vi "GetFilterList.vi"(11 "Templates":refnum<class "MetaDataObj.lvclass">[](array[class])) -> (3 "Filters":string[](array[string]))   [LabVIEW 2016, in "NI_NPW_Filters.lvlib"]
uses:
  <resource>/dialog/NewProjectWizard/Filters/NI_NPW_Filters.lvlib
  <resource>/dialog/NewProjectWizard/MetaDataObj/MetaDataObj.lvclass
  <resource>/dialog/NewProjectWizard/MetaDataObj/Accessors/Read Filters.vi
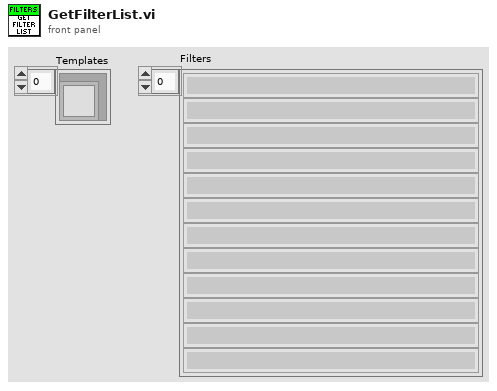
[diagram p1: front panel]
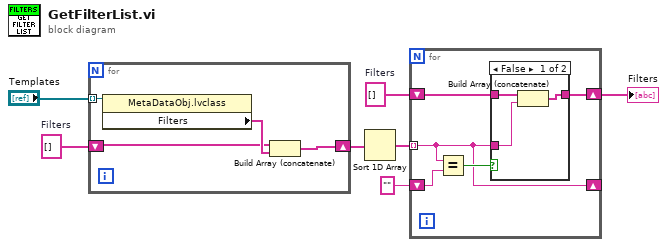
[diagram p0: block diagram]
diagram:
  w4 = string[] []  # Filters
  w6 = string[] []  # Filters
  n1 = for {
    tunnel: "Templates" -> [w11] mode=indexing
    shift-right: [w8] -> w5
    shift-left: w6 -> [w9]
    n2 = property class="MetaDataObj.lvclass"(reference=w11) -> ("Filters"=w10:string[])  [unwired: 1 in, 2 out]
    n3 = Build Array (concatenate)(w9, w10) -> (w8:string[])
  }
  n4 = Sort 1D Array(array=w5) -> (sorted array=w3:string[])
  n5 = for {
    shift-right: [w13] -> w1
    shift-left: w4 -> [w14]
    tunnel: w3 -> [w12] mode=indexing
    shift-right: [w12] -> _
    shift-left: "" ("String") -> [w15]
    n6 = Equal?(x=w12, y=w15) -> (x = y?=w16:bool)
    n7 = case shown="False" w16 {
      tunnel: w14 -> [w18 w20]
      tunnel: [w19 w20] -> w13
      tunnel: w12 -> [w17 _]
      frame False {
        n8 = Build Array (concatenate)(w18, w17) -> (w19:string[])
      }
      frame True {
      }
    }
  }
  "Filters" <- w1
